vi "IOtest.vi"() -> ()   [LabVIEW 2019]
uses:
  <vilib>/Utility/file.llb/Write Delimited Spreadsheet (DBL).vi
panel:
  out "size(s)":i32[](array[numeric])
  out "Numeric":i32
  in  "stop":bool
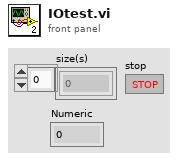
[diagram p1: front panel]
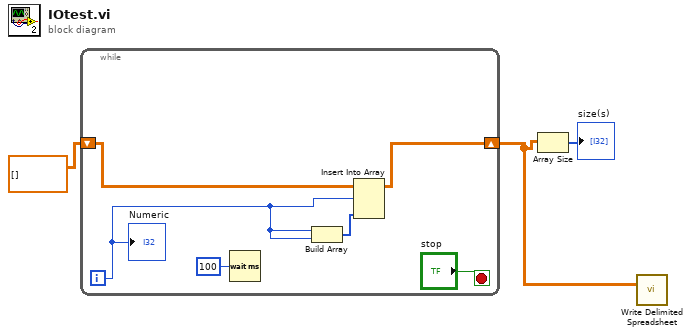
[diagram p0: block diagram]
diagram:
  n1 = while {
    shift-right: [w8] -> w2
    shift-left: dbl[][] [] ("array") -> [w7]
    i -> [w5]
    stop <- "stop" stop-if-true
    n2 = Wait (ms)(milliseconds to wait=u32 100) -> ()  [unwired: 1 out]
    n3 = Build Array(w5, w5) -> (w4:i32[])
    n4 = Insert Into Array(array=w7, index (row)=w5, new element=w4) -> (w8:dbl[][])  [unwired: 1 in]
    "Numeric" <- w5
  }
  n5 = Array Size(array=w2) -> (size(s)=→"size(s)":i32[])
  n6 = call-poly <vilib>:"Write Delimited Spreadsheet.vi"("2D data"=w2) -> ()  [unwired: 13 in, 2 out]
